vi "SpectToAllWaveform.vi"() -> ()   [LabVIEW 2014]
uses:
  <vilib>/Utility/file.llb/Read From Spreadsheet File (DBL).vi
panel:
  out "File name":string
  out "N Files":i32
  out "XY Graph array":cluster{"Array":dbl[], "Array":dbl[]}[][](array[cluster])
  out "XY Graph":cluster{dbl[], dbl[]}[](graph)
  out "Total Specs":i32=105
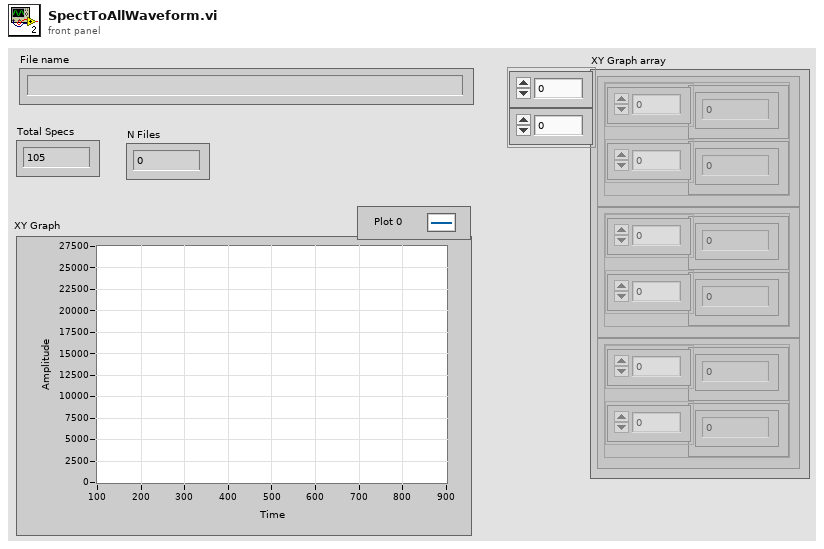
[diagram p1: front panel]
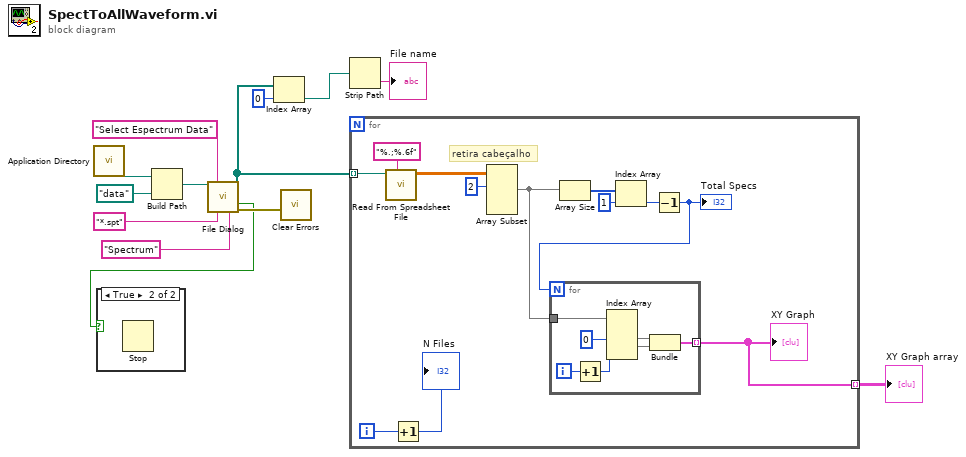
[diagram p0: block diagram]
diagram:
  n1 = call <vilib>:"Application Directory.vi"() -> ("Application Directory"=w9:path)
  n2 = Build Path(base path=w9, name or relative path=path "data") -> (appended path=w8:path)
  n3 = call "File Dialog"("start path"=w8, "prompt"="Select Espectrum Data", "pattern (all files)"="*.spt", "pattern label"="Spectrum") -> ("selected paths"=w4:path[], "cancelled"=w6:bool, "error out"=w7:errorcluster)  [unwired: 8 in, 1 out]
  n4 = case shown="True" w6 {
    frame False {
    }
    frame True {
      n5 = Stop() -> ()  [unwired: 1 in]
    }
  }
  n6 = Index Array(array=w4, index=0) -> (element=w2:path)
  n7 = call <vilib>:"Clear Errors.vi"("error in (no error)"=w7) -> ()  [unwired: 5 in, 2 out]
  n8 = Strip Path(path=w2) -> (name=→"File name":string)  [unwired: 1 out]
  n9 = for {
    tunnel: w4 -> [w17] mode=indexing
    tunnel: [w16] -> w5 mode=indexing
    i -> [w15]
    # "retira cabeçalho"
    n10 = call-poly <vilib>:"Read From Spreadsheet File.vi"("format (%.3f)"="%.;%.6f", "file path (dialog if empty)"=w17) -> ("all rows"=w23:dbl[][])  [unwired: 5 in, 4 out]
    n11 = Increment(x=w15) -> (x+1=→"N Files":i32)
    n12 = Array Subset(array=w23, index (row)=2 ("index")) -> (w18:dbl[][])  [unwired: 3 in]
    n13 = Array Size(array=w18) -> (size(s)=w22:i32[])
    n14 = Index Array(array=w22, index=1) -> (element=w20:i32)
    n15 = Decrement(x=w20) -> (x-1=w19:i32)
    "Total Specs" <- w19
    n16 = for {
      N: w19 -> [_]
      tunnel: w18 -> [w32]
      tunnel: [w28] -> w16 mode=indexing
      i -> [w27]
      n17 = Increment(x=w27) -> (x+1=w26:i32)
      n18 = Index Array(array=w32, index (col) #1=0 ("index (row)"), index (col) #2=w26) -> (element #1=w30:dbl[], element #2=w29:dbl[])  [unwired: 2 in]
      n19 = Bundle(w30, w29) -> (w28:cluster{dbl[], dbl[]})  [unwired: 1 in]
    }
    "XY Graph" <- w16
  }
  "XY Graph array" <- w5
